vi "TEST CDAQ.vi"() -> ()   [LabVIEW 2017]
uses:
  <vilib>/DAQmx/write.llb/DAQmx Write (Digital 2D Bool NChan 1Samp NLine).vi
  <vilib>/DAQmx/create/channels.llb/DAQmx Create Channel (DO-Digital Output).vi
  <vilib>/DAQmx/miscellaneous.llb/DAQmx Fill In Error Info.vi
panel:
  in  "data":bool[][](array[boolean])
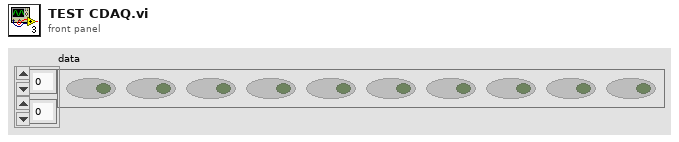
[diagram p1: front panel]
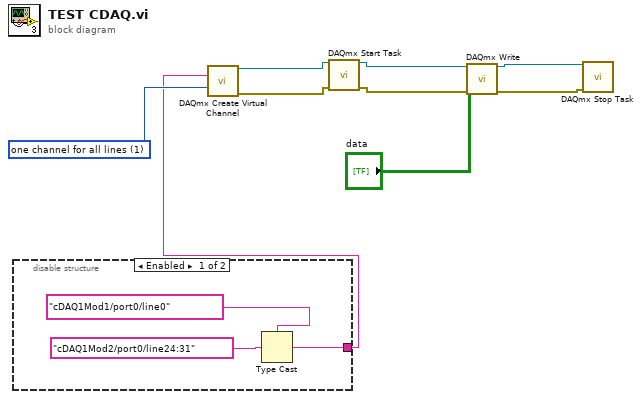
[diagram p0: block diagram]
diagram:
  w3 = 1 items=["one channel for each line", "one channel for all lines"] ("line grouping")
  n1 = disable-structure shown="Enabled" {
    disable-tunnel: [w10 _] -> w2
    frame Enabled {
      n2 = Type Cast(type=tag "cDAQ1Mod1/port0/line0" ("lines"), x="cDAQ1Mod2/port0/line24:31") -> (*(type *) &x=w10:tag)
    }
    frame Disabled {
    }
  }
  n3 = call-poly <vilib>:"DAQmx Create Virtual Channel.vi"("lines"=w2, "line grouping"=w3) -> ("task out"=w9:refnum<k21>, "error out"=w8:errorcluster)  [unwired: 12 in]
  n4 = call <vilib>:"DAQmx Start Task.vi"("task/channels in"=w9, "error in"=w8) -> ("task out"=w7:refnum<k21>, "error out"=w6:errorcluster)  [unwired: 12 in]
  n5 = call-poly <vilib>:"DAQmx Write.vi"("task/channels in"=w7, "data"="data", "error in"=w6) -> ("task out"=w5:refnum<k21>, "error out"=w4:errorcluster)  [unwired: 10 in, 1 out]
  n6 = call <vilib>:"DAQmx Stop Task.vi"("task/channels in"=w5, "error in"=w4) -> ()  [unwired: 12 in, 2 out]
